vi "ATF-Pump-DO cluster to data.vi"(11 "output cluster":T1) -> (1 "Numeric":dbl, 2 "Component ID":string, 3 "Boolean":bool, 5 "Sequence":string)   [LabVIEW 2022 SP3]
doc: "This is an exclusive vi created to get the cluster data to Boolean ,String and Numeric"
panel:
  out "length":i32
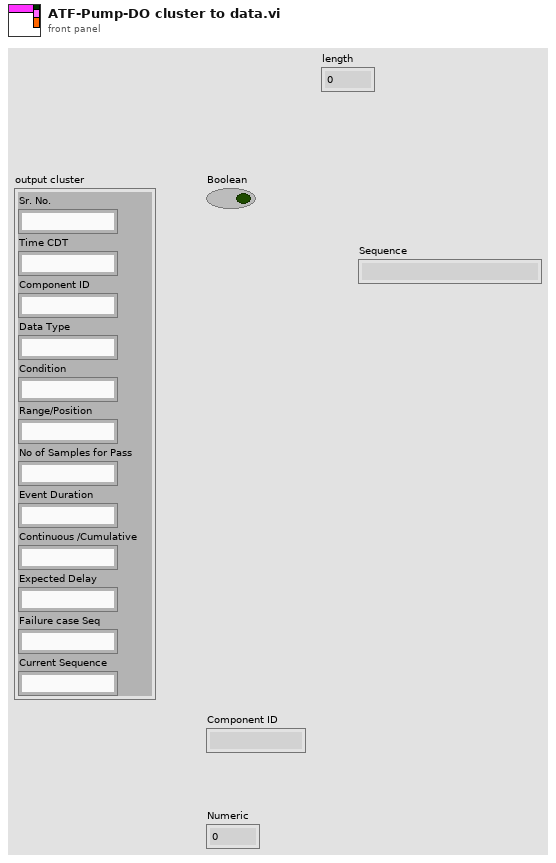
[diagram p1: front panel]
types:
  T1 = cluster{"Sr. No.":string, "Time CDT":string, "Component ID":string, "Data Type":string, "Condition":string, "Range/Position":string, "No of Samples for Pass":string, "Event Duration":string, "Continuous /Cumulative":string, "Expected Delay":string, "Failure case Seq":string, "Current Sequence":string}
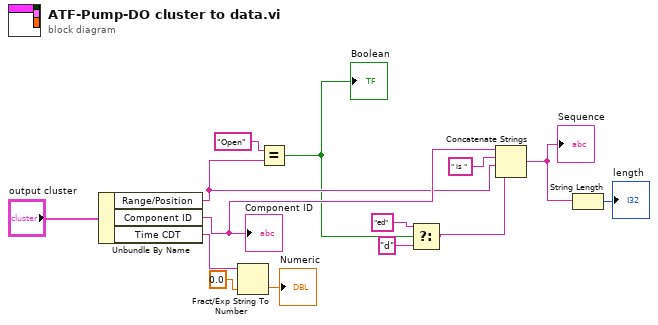
[diagram p0: block diagram]
diagram:
  n1 = Unbundle By Name("output cluster") -> ("Range/Position"=w7:string, "Component ID"=w9:string, "Time CDT"=w11:string)
  "Component ID" <- w9
  n2 = Fract/Exp String To Number(string=w11, default (0 dbl)=0.0 ("CDT")) -> (number=→"Numeric":dbl)  [unwired: 2 in, 1 out]
  n3 = Equal?(x="Open" ("y"), y=w7) -> (x = y?=w6:bool)
  "Boolean" <- w6
  n4 = Select(t="ed" ("string"), s=w6, f="d") -> (s? t:f=w3:string)
  n5 = Concatenate Strings(w9, " is " ("string"), w7, w3) -> (w2:string)
  "Sequence" <- w2
  n6 = String Length(string=w2) -> (length=→"length":i32)
